vi "DivideDownVectors.vi"(1 "Frame Prams":cluster{"Divide By":u8, "frames":i32}, 4 "Total Lines":i32) -> (6 "task out":refnum<k21>, 7 "error out":errorcluster)   [LabVIEW 2022 SP3]
uses:
  <vilib>/DAQmx/create/channels.llb/DAQmx Create Channel (CO-Pulse Generation-Ticks).vi
  <vilib>/DAQmx/configure/trigger.llb/DAQmx Start Trigger (None).vi
  <vilib>/DAQmx/configure/timing.llb/DAQmx Timing (Implicit).vi
panel:
  in  "error in":errorcluster
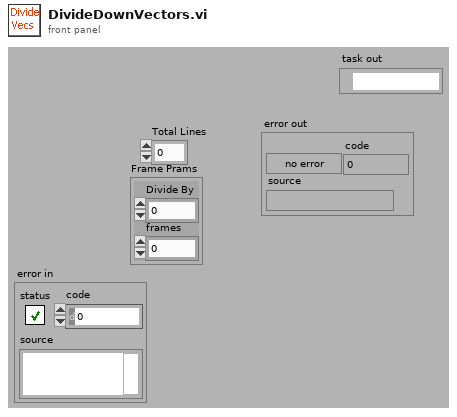
[diagram p1: front panel]
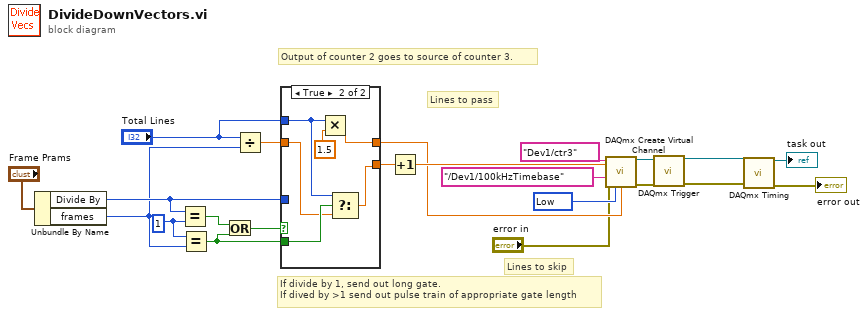
[diagram p0: block diagram]
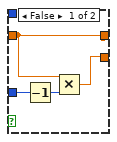
[diagram p2: hidden frame]
diagram:
  w7 = 10214 items=["High"=10192, "Low"=10214] ("idle state")
  w15 = 1
  # "Output of counter 2 goes to source of counter 3."
  # "Lines to skip"
  # "Lines to pass"
  # "If divide by 1, send out long gate.\nIf dived by >1 send out pulse train of appropriate gate length"
  n1 = Unbundle By Name("Frame Prams") -> ("Divide By"=w21:u8, "frames"=w16:i32)
  n2 = Equal?(x=w21, y=w15) -> (x = y?=w18:bool)
  n3 = Equal?(x=w15, y=w16) -> (x = y?=w14:bool)
  n4 = Or(x=w18, y=w14) -> (x .or. y?=w17:bool)
  n5 = Divide(x="Total Lines", y=w16) -> (x/y=w20:dbl)
  n6 = case shown="True" w17 {
    tunnel: w20 -> [w24 w27]
    tunnel: [w24 w32] -> w10
    tunnel: [w23 w28] -> w13
    tunnel: w21 -> [w26 _]
    tunnel: "Total Lines" -> [_ w29]
    tunnel: w14 -> [_ w30]
    frame False {
      n7 = Decrement(x=w26) -> (x-1=w25:u8)
      n8 = Multiply(x=w24, y=w25) -> (x*y=w23:dbl)
    }
    frame True {
      n9 = Multiply(x=w29, y=1.5) -> (x*y=w32:dbl)
      n10 = Select(t=w29, s=w30, f=w27) -> (s? t:f=w28:dbl)
    }
  }
  n11 = Increment(x=w13) -> (x+1=w11:dbl)
  n12 = call-poly <vilib>:"DAQmx Create Virtual Channel.vi"("high ticks"=w11, "counter"=tag "Dev1/ctr3", "source of ticks"=tag "/Dev1/100kHzTimebase", "error in"="error in", "idle state"=w7, "initial delay"=w10) -> ("task out"=w6:refnum<k21>, "error out"=w5:errorcluster)  [unwired: 3 in, 5 out]
  n13 = call-poly <vilib>:"DAQmx Trigger.vi"("task/channels in"=w6, "error in"=w5) -> ("task out"=w4:refnum<k21>, "error out"=w3:errorcluster)  [unwired: 12 out]
  n14 = call-poly <vilib>:"DAQmx Timing.vi"("task/channels in"=w4, "error in"=w3) -> ("task out"=→"task out":refnum<k21>, "error out"=→"error out":errorcluster)  [unwired: 3 in, 9 out]
